vi "xbee_switch_mode.vi"(8 "error in":errorcluster, 10 "Global":bool, 11 "com in":refnum<visa-resource-name>) -> (0 "error out":errorcluster, 3 "com out":refnum<visa-resource-name>)   [LabVIEW 2012]
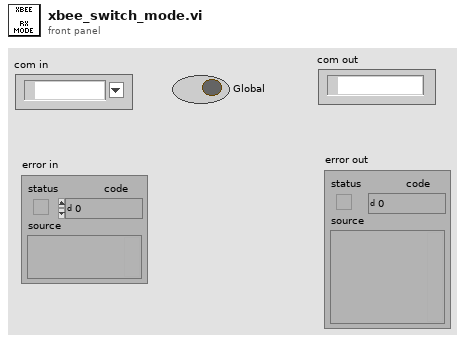
[diagram p1: front panel]
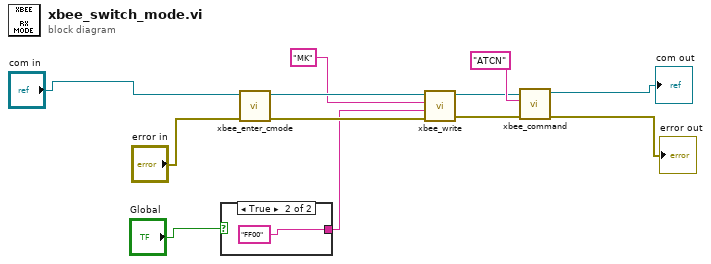
[diagram p0: block diagram]
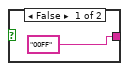
[diagram p2: hidden frame]
diagram:
  n1 = case shown="True" "Global" {
    tunnel: ["00FF" "FF00"] -> w7
    frame False {
    }
    frame True {
    }
  }
  n2 = call "xbee_enter_cmode.vi"("error in (no error)"="error in", "COM in"="com in") -> ("error out"=w10:errorcluster, "COM out"=w11:refnum<visa-resource-name>)  [unwired: 8 in]
  n3 = call "xbee_write.vi"("error in"=w10, "value"=w7, "command"="MK", "com in"=w11) -> ("error out"=w4:errorcluster, "com out"=w5:refnum<visa-resource-name>)  [unwired: 6 in]
  n4 = call "xbee_command.vi"("error in (no error)"=w4, "command"="ATCN", "COM in"=w5) -> ("error out"=→"error out":errorcluster, "COM out"=→"com out":refnum<visa-resource-name>)  [unwired: 6 in, 1 out]
